vi "PSTR-Show Legend.vi"(0 "ListBox in":refnum<vi>, 5 "Data":T1) -> ()   [LabVIEW 2020]
uses:
  Typedefs/PSTR-Data.ctl
  Typedefs/PSTR-Model Fit.ctl
  Typedefs/PSTR-Fit Parameters.ctl
panel:
  # "NF x NL x 2 x Npts"
  # "NF x NL x Npts"
  # "NF x NL"
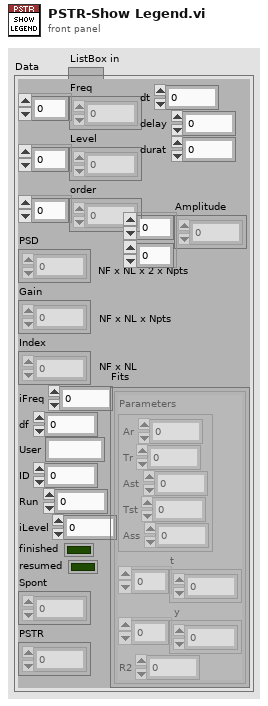
[diagram p1: front panel]
types:
  T1 = typedef "PSTR-Data.ctl" = cluster{"Freq":dbl[], "Level":dbl[], "order":i32[], "PSD":dbl[][][][], "Gain":dbl[][][], "Index":dbl[][], "iFreq":i32, "df":dbl, "User":string, "ID":i32, "Run":i32, "iLevel":i32, "finished":bool, "resumed":bool, "Spont":dbl[][], "PSTR":dbl[][][], "dt":dbl, "delay":dbl, "durat":dbl, "Fits":T2[][], "Amplitude":dbl[][]}
  T2 = typedef "PSTR-Model Fit.ctl" = cluster{"Parameters":T3, "t":dbl[], "y":dbl[], "R2":dbl}
  T3 = typedef "PSTR-Fit Parameters.ctl" = cluster{"Ar":dbl, "Tr":dbl, "Ast":dbl, "Tst":dbl, "Ass":dbl}
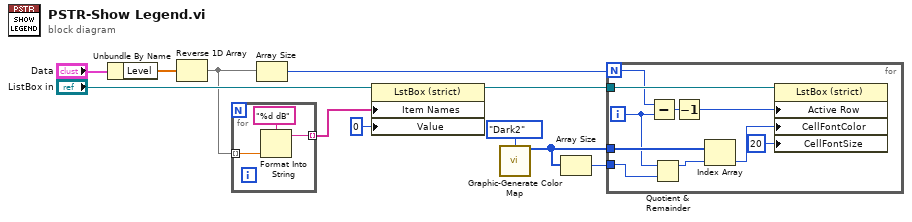
[diagram p0: block diagram]
diagram:
  n1 = Unbundle By Name("Data") -> ("Level"=w7:dbl[])
  n2 = Reverse 1D Array(array=w7) -> (reversed array=w4:dbl[])
  n3 = for {
    tunnel: w4 -> [w13] mode=indexing
    tunnel: [w12] -> w11 mode=indexing
    n4 = Format Into String(format string="%d dB", w13) -> (resulting string=w12:string)  [unwired: 2 in, 1 out]
  }
  n5 = Array Size(array=w4) -> (size(s)=w6:i32)
  n6 = property on="Property Node" class="LstBox (strict)"(reference="ListBox in", "Item Names"=w11, "Value"=0) -> (reference out=w8:refnum<vi>)  [unwired: 1 in, 1 out]
  n7 = call "Graphic-Generate Color Map.vi"("Map"=enum16{"User", "Prism", "Kelly", "Dark2"}."Dark2") -> ("Colors"=w3:u32[])  [unwired: 14 in]
  n8 = Array Size(array=w3) -> (size(s)=w2:i32)
  n9 = for {
    N: w6 -> [w20]
    tunnel: w8 -> [w24]
    tunnel: w3 -> [w23]
    tunnel: w2 -> [w17]
    i -> [w15]
    n10 = Subtract(x=w20, y=w15) -> (x-y=w19:i32)
    n11 = Quotient & Remainder(x=w15, y=w17) -> (x-y*floor(x/y)=w16:i32)  [unwired: 1 out]
    n12 = Decrement(x=w19) -> (x-1=w18:i32)
    n13 = Index Array(array=w23, index=w16) -> (element=w22:u32)
    n14 = property on="Property Node" class="LstBox (strict)"(reference=w24, "Active Row"=w18, "CellFontColor"=w22, "CellFontSize"=u32 20 ("Active Row:Cell Font:Size")) -> ()  [unwired: 1 in, 2 out]
  }
